vi "SHUTDOWN.vi"(0 "refnum in":refnum<vi>, 2 "Option":enum16{"None", "SAVE", "NOSAVE"}(ring), 11 "error in":errorcluster) -> (4 "refnum out":refnum<vi>, 6 "Data":T1, 15 "error out":errorcluster)   [LabVIEW 2020]
uses:
  SubVIs/Controls/redis-data.ctl
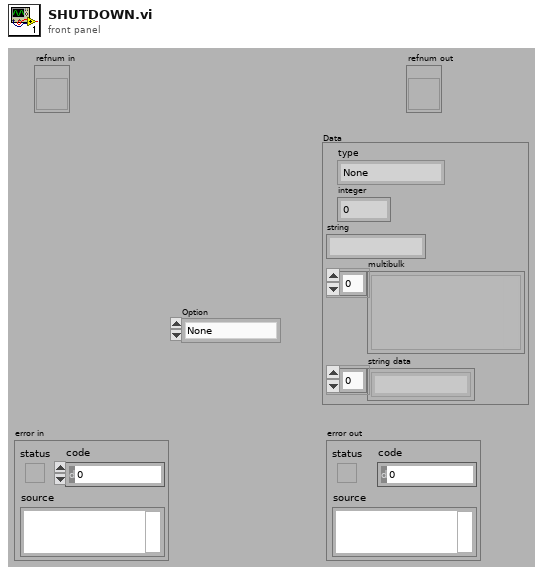
[diagram p1: front panel]
types:
  T1 = typedef "redis-data.ctl" = cluster{"type":enum16{"None", "Error", "Status", "Nil", "Integer", "String", "Multibulk"}, "integer":i64, "string":string, "multibulk":variant[], "string data":string[]}
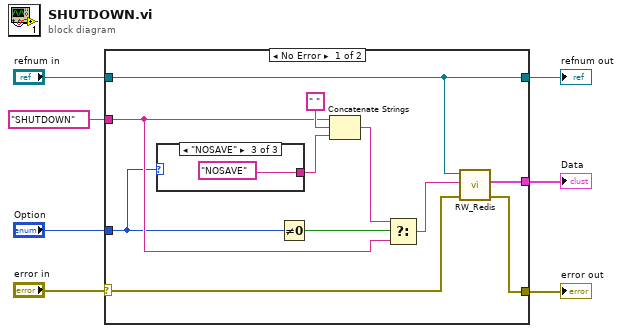
[diagram p0: block diagram]
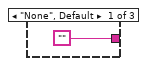
[diagram p2: hidden frame]
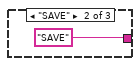
[diagram p3: hidden frame]
diagram:
  n1 = case shown="No Error" "error in" {
    selector: "error in" -> [w18 w23]
    tunnel: "SHUTDOWN" -> [w9 _]
    tunnel: "refnum in" -> [w15 w22]
    tunnel: [w17 w23] -> w5
    tunnel: [w16 _] -> w2
    tunnel: [w15 w22] -> w4
    tunnel: "Option" -> [w8 _]
    frame No Error {
      n2 = case shown="\"NOSAVE\"" w8 {
        tunnel: ["" "SAVE" "NOSAVE"] -> w12
        frame "None", Default {
        }
        frame "SAVE" {
        }
        frame "NOSAVE" {
        }
      }
      n3 = Not Equal To 0?(x=w8) -> (x != 0?=w14:bool)
      n4 = Concatenate Strings(w9, " ", w12) -> (w11:string)
      n5 = Select(t=w11, s=w14, f=w9) -> (s? t:f=w10:string)
      n6 = call "RW_Redis.vi"("error in"=w18, "command"=w10, "refnum"=w15) -> ("error out"=w17:errorcluster, "Data"=w16:T1)  [unwired: 7 in]
    }
    frame Error {
    }
  }
  "error out" <- w5
  "Data" <- w2
  "refnum out" <- w4
